vi "Create DO Channel.vi"(8 "error in (no error)":errorcluster, 11 "DO Channel Setting":T1={"DO Channel"=["6363/port1/line0", "6363/port1/line1", "6363/port1/line2", "6363/port1/line3"]}) -> (0 "error out":errorcluster, 3 "DO_Task":refnum<k21>)   [LabVIEW 2016, in "DAQ Hardware.lvlib"]
uses:
  DAQ Hardware.lvlib
  DO Channel Setting.ctl
  <vilib>/DAQmx/create/channels.llb/DAQmx Create Channel (DO-Digital Output).vi
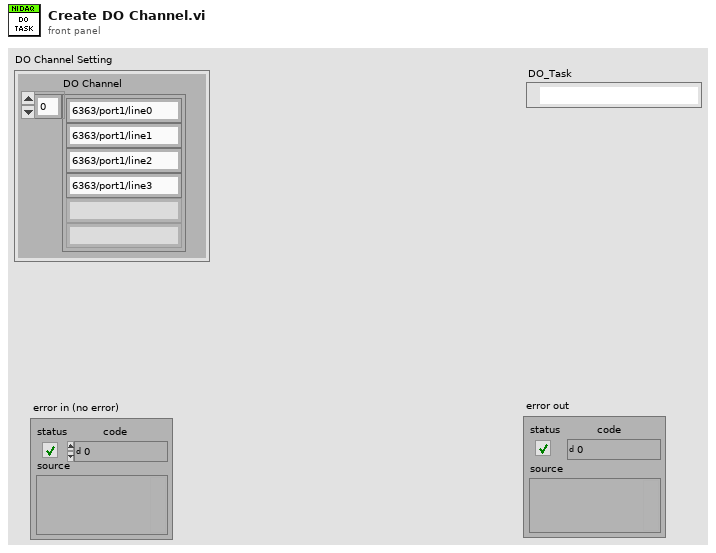
[diagram p1: front panel]
types:
  T1 = typedef "DAQ Hardware.lvlib/DO Channel Setting.ctl" = cluster{"DO Channel":string[]}
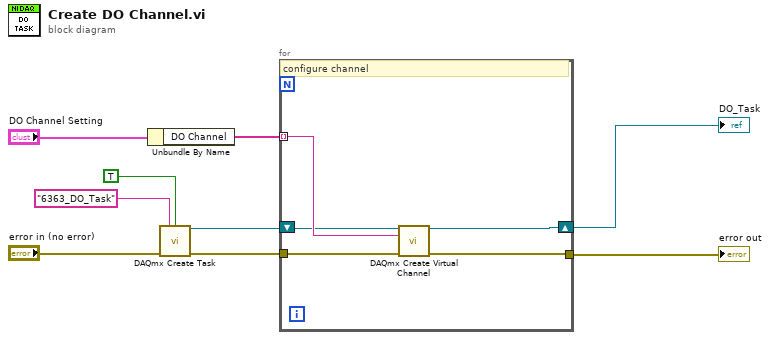
[diagram p0: block diagram]
diagram:
  n1 = Unbundle By Name("DO Channel Setting") -> ("DO Channel"=w4:string[])
  n2 = call <vilib>:"DAQmx Create Task.vi"("new task name"="6363_DO_Task" ("name to assign"), "auto cleanup"=TRUE, "error in"="error in (no error)") -> ("task out"=w2:refnum<k21>, "error out"=w6:errorcluster)  [unwired: 11 in]
  n3 = for {
    tunnel: w6 -> [w14]
    tunnel: w4 -> [w11] mode=indexing
    tunnel: [w13] -> w9
    shift-right: [w12] -> w1
    shift-left: w2 -> [w10]
    # "configure channel"
    n4 = call-poly <vilib>:"DAQmx Create Virtual Channel.vi"("task in"=w10, "Lines"=w11, "error in"=w14) -> ("task out"=w12:refnum<k21>, "error out"=w13:errorcluster)  [unwired: 11 in]
  }
  "error out" <- w9
  "DO_Task" <- w1
